vi "array_portion (SubVI).vi"(9 "Starting Point":i32, 10 "Portion Duration":i32, 11 "Input Array":dbl[](array[numeric])) -> (2 "Remain":dbl[](array[numeric]), 3 "Portion":dbl[](array[numeric]))   [LabVIEW 2012]
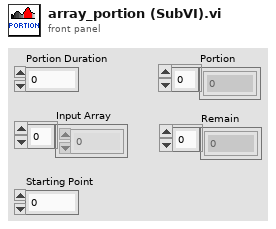
[diagram p1: front panel]
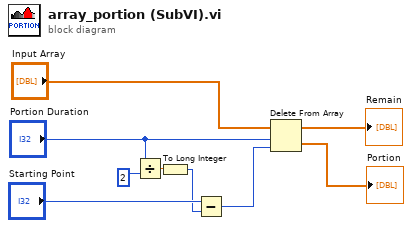
[diagram p0: block diagram]
diagram:
  n1 = Divide(x="Portion Duration", y=2) -> (x/y=w9:dbl)
  n2 = To Long Integer(number=w9) -> (32bit integer=w6:i32)
  n3 = Subtract(x="Starting Point", y=w6) -> (x-y=w4:i32)
  n4 = Delete From Array(array="Input Array", length="Portion Duration", index=w4) -> (deleted portion=→"Portion":dbl[], array with subset deleted=→"Remain":dbl[])
